vi "test_1_1.vi"() -> ()   [LabVIEW 2010]
panel:
  in  "几个":i32
  out "显示":i32[](array[numeric])
  in  "输入":i32[][](array[numeric])
  in  "关闭":bool
  in  "开始":bool
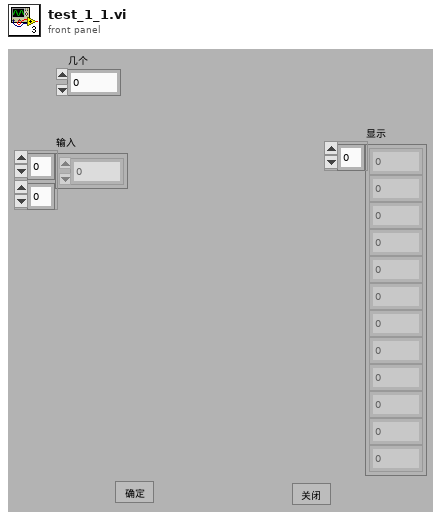
[diagram p1: front panel]
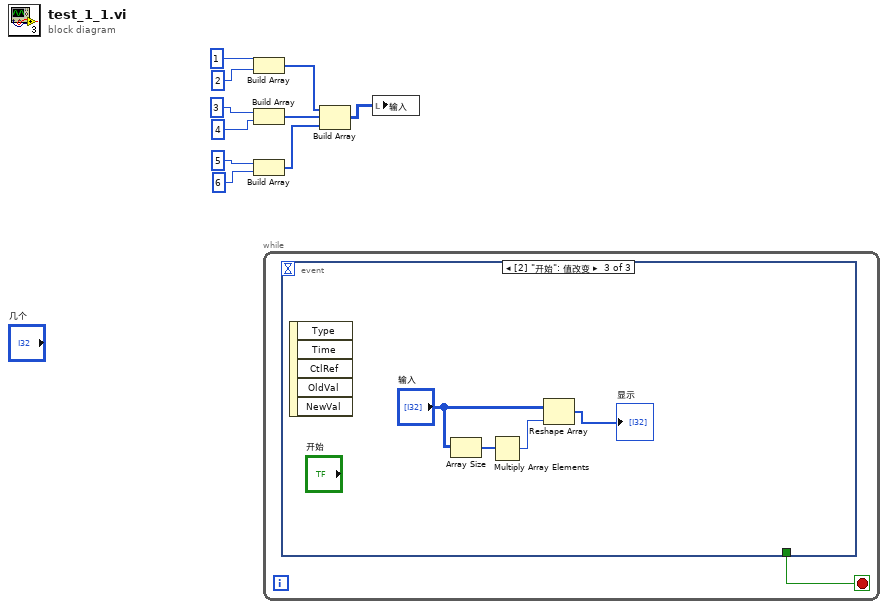
[diagram p0: block diagram]
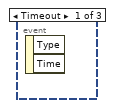
[diagram p2: hidden frame]
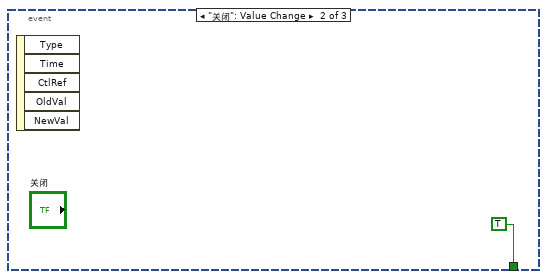
[diagram p3: hidden frame]
diagram:
  n1 = Build Array(1 ("数值"), 2 ("数值")) -> (w4:i32[])
  n2 = Build Array(3 ("数值"), 4 ("数值")) -> (w3:i32[])
  n3 = Build Array(5 ("数值"), 6 ("数值")) -> (w2:i32[])
  n4 = while {
    stop <- w11 stop-if-true
    n5 = event shown="[2] \"开始\": 值改变" {
      selector: _ -> [_ _ _]
      dyn-events: _ -> [_ _ _]
      timeout: _ -> [_ _ _]
      tunnel: [_ TRUE _] -> w11
      event Timeout {
        n6 = event-data() -> ()  [unwired: 1 in, 2 out]
      }
      event "关闭": Value Change {
        n7 = event-data() -> ()  [unwired: 1 in, 5 out]
      }
      event "开始": Value Change {
        n8 = event-data() -> ()  [unwired: 1 in, 5 out]
        n9 = Array Size(array="输入") -> (size(s)=w14:i32[])
        n10 = Multiply Array Elements(1:w14) -> (0:w13:i32)
        n11 = Reshape Array("输入", w13) -> (→"显示":i32[])
      }
    }
  }
  n12 = Build Array(w4, w3, w2) -> (w1:i32[][])
  n13 = local write "输入"(w1) -> ()
